vi "ConfigUSB.vi"(2 "Purge?":bool) -> (5 "Status":bool, 6 "Handle ChA":u32, 7 "Description ChA":string, 9 "Handle ChB 2":u32, 10 "Description ChB":string)   [LabVIEW 2010]
panel:
  out "Device Info List":T1(array[cluster]) {"FT_Handle" format="%.0x"; "LocID" format="%.0x"; "PID" format="%.0x"; "VID" format="%.0x"; "Type" items=["FT232B-FT245B", "FT8U232AM-FT8U245AM", "FT8U100AX", "UNKNOWN", "FT2232", "FT232R", "FT2232H", "FT4232H"]}
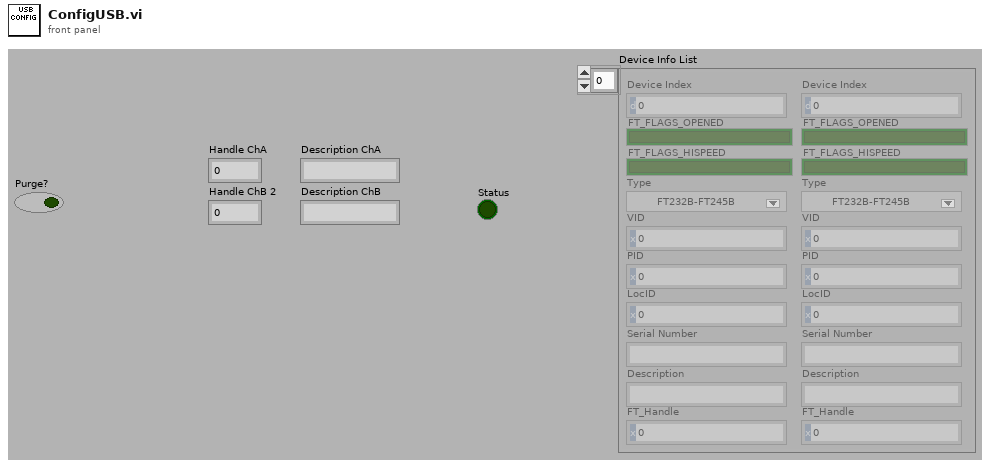
[diagram p1: front panel]
types:
  T1 = cluster{"Device Index":u32, "FT_FLAGS_OPENED":bool, "FT_FLAGS_HISPEED":bool, "Type":u32, "VID":u32, "PID":u32, "LocID":i32, "Serial Number":string, "Description":string, "FT_Handle":u32}[]
  T2 = cluster{"Device Index":u32, "FT_FLAGS_OPENED":bool, "FT_FLAGS_HISPEED":bool, "Type":u32, "VID":u32, "PID":u32, "LocID":i32, "Serial Number":string, "Description":string, "FT_Handle":u32}
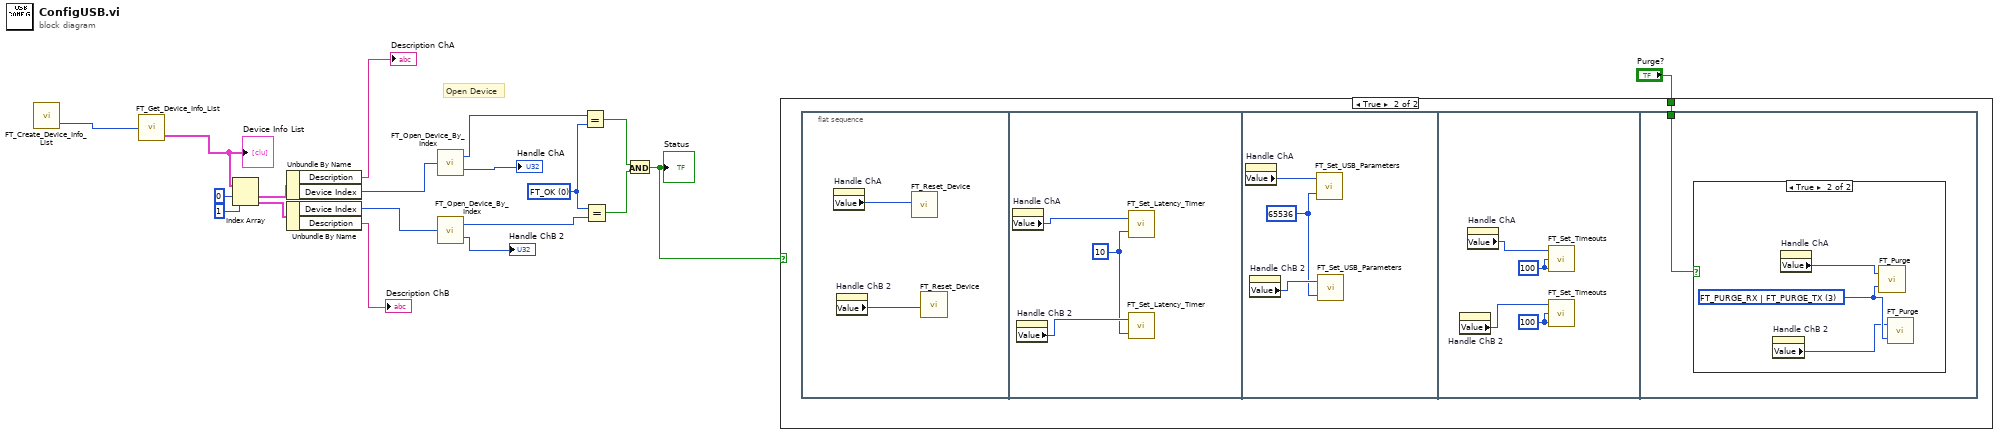
[diagram p0: block diagram]
diagram:
  w17 = u32 0 items=["FT_OK", "FT_INVALID_HANDLE", "FT_DEVICE_NOT_FOUND", "FT_DEVICE_NOT_OPENED", "FT_IO_ERROR", "FT_INSUFFICIENT_RESOURCES", "FT_INVALID_PARAMETER", "FT_INVALID_BAUD_RATE", "FT_DEVICE_NOT_OPENED_FOR_ERASE", "FT_DEVICE_NOT_OPENED_FOR_WRITE", "FT_FAILED_TO_WRITE_DEVICE", "FT_EEPROM_READ_FAILED", "FT_EEPROM_WRITE_FAILED", "FT_EEPROM_ERASE_FAILED", "FT_EEPROM_NOT_PRESENT", "FT_EEPROM_NOT_PROGRAMMED", "FT_INVALID_ARGS", "FT_NOT_SUPPORTED", "FT_OTHER_ERROR"] ("FT_Status")
  # "Open Device"
  n1 = call "FT_Create_Device_Info_List.vi"() -> ("Number of Devices"=w6:u32)  [unwired: 1 out]
  n2 = call "FT_Get_Device_Info_List.vi"("Number Of Devices"=w6) -> ("Device Info List"=w7:T1)  [unwired: 1 out]
  "Device Info List" <- w7
  n3 = Index Array(array=w7, index #1=0 ("index"), index #2=1 ("index")) -> (element #1=w8:T2, element #2=w11:T2)
  n4 = Unbundle By Name(w8) -> ("Description"=→"Description ChA":string, "Device Index"=w2:u32)
  n5 = Unbundle By Name(w11) -> ("Device Index"=w12:u32, "Description"=→"Description ChB":string)
  n6 = call "FT_Open_Device_By_Index.vi"("Device Index"=w2) -> ("FT_Status"=w15:u32, "Handle"=→"Handle ChA":u32)
  n7 = call "FT_Open_Device_By_Index.vi"("Device Index"=w12) -> ("FT_Status"=w16:u32, "Handle"=→"Handle ChB 2":u32)
  n8 = Equal?(x=w15, y=w17) -> (x = y?=w18:bool)
  n9 = Equal?(x=w17, y=w16) -> (x = y?=w19:bool)
  n10 = And(x=w18, y=w19) -> (x .and. y?=w5:bool)
  "Status" <- w5
  n11 = case shown="True" w5 {
    tunnel: "Purge?" -> [_ w20]
    frame False {
    }
    frame True {
      n12 = flat-sequence {
        tunnel: w20 -> [w33]
        frame #0 {
          n13 = property on="Handle ChA" class="DigNum (strict)"() -> ("Value"=w21:u32)  [unwired: 2 in, 2 out]
          n14 = property on="Handle ChB 2" class="DigNum (strict)"() -> ("Value"=w22:u32)  [unwired: 2 in, 2 out]
          n15 = call "FT_Reset_Device.vi"("Handle"=w21) -> ()  [unwired: 1 out]
          n16 = call "FT_Reset_Device.vi"("Handle"=w22) -> ()  [unwired: 1 out]
        }
        frame #1 {
          w23 = u8 10 ("Latency Timer Value")
          n17 = property on="Handle ChA" class="DigNum (strict)"() -> ("Value"=w25:u32)  [unwired: 2 in, 2 out]
          n18 = property on="Handle ChB 2" class="DigNum (strict)"() -> ("Value"=w24:u32)  [unwired: 2 in, 2 out]
          n19 = call "FT_Set_Latency_Timer.vi"("Latency Timer Value"=w23, "Handle"=w25) -> ()  [unwired: 1 out]
          n20 = call "FT_Set_Latency_Timer.vi"("Latency Timer Value"=w23, "Handle"=w24) -> ()  [unwired: 1 out]
        }
        frame #2 {
          w26 = u32 65536 ("In Transfer Size")
          n21 = property on="Handle ChA" class="DigNum (strict)"() -> ("Value"=w27:u32)  [unwired: 2 in, 2 out]
          n22 = property on="Handle ChB 2" class="DigNum (strict)"() -> ("Value"=w28:u32)  [unwired: 2 in, 2 out]
          n23 = call "FT_Set_USB_Parameters.vi"("In Transfer Size"=w26, "Handle"=w27) -> ()  [unwired: 1 out]
          n24 = call "FT_Set_USB_Parameters.vi"("In Transfer Size"=w26, "Handle"=w28) -> ()  [unwired: 1 out]
        }
        frame #3 {
          w29 = u32 100 ("Read Timeout")
          w30 = u32 100 ("Read Timeout")
          n25 = property on="Handle ChB 2" class="DigNum (strict)"() -> ("Value"=w32:u32)  [unwired: 2 in, 2 out]
          n26 = property on="Handle ChA" class="DigNum (strict)"() -> ("Value"=w31:u32)  [unwired: 2 in, 2 out]
          n27 = call "FT_Set_Timeouts.vi"("Write Timeout"=w29, "Read Timeout"=w29, "Handle"=w31) -> ()  [unwired: 1 out]
          n28 = call "FT_Set_Timeouts.vi"("Write Timeout"=w30, "Read Timeout"=w30, "Handle"=w32) -> ()  [unwired: 1 out]
        }
        frame #4 {
          n29 = case shown="True" w33 {
            frame False {
            }
            frame True {
              w36 = u32 3 items=["FT_PURGE_RX"=1, "FT_PURGE_TX"=2, "FT_PURGE_RX | FT_PURGE_TX"=3] ("Purge Flags")
              n30 = property on="Handle ChB 2" class="DigNum (strict)"() -> ("Value"=w35:u32)  [unwired: 2 in, 2 out]
              n31 = property on="Handle ChA" class="DigNum (strict)"() -> ("Value"=w34:u32)  [unwired: 2 in, 2 out]
              n32 = call "FT_Purge.vi"("Purge Flags"=w36, "Handle"=w34) -> ()  [unwired: 1 out]
              n33 = call "FT_Purge.vi"("Purge Flags"=w36, "Handle"=w35) -> ()  [unwired: 1 out]
            }
          }
        }
      }
    }
  }
